vi "Autonomous Independent.vi"() -> ()   [LabVIEW 2014]
doc: "This VI is called when autonomous begins, and will automatically be terminated when autonomous ends. You can carry out timed or sensor driven robot movement independently without needing to return to the caller."
uses:
  <vilib>/Rock Robotics/WPI/DriverStation/WPI_DriverStationRobotMode2.ctl
  <vilib>/Rock Robotics/WPI/RobotDrive/WPI_RobotDriveGetSetRefNum.vi
  <vilib>/Rock Robotics/Network Tables/SD Write Numeric Array.vi
  <vilib>/Rock Robotics/WPI/RobotDrive/WPI_RobotDriveArcadeDrive_Standard(NoSaturation).vi
panel:
  out "Current Movement, for debugging":T1 {"Y Joystick Value" scale=1.0..-1.0; "X Joystick Value" scale=-1.0..1.0}
  in  "Array of robot movements":T2(array[cluster]) {"Y Joystick Value" scale=1.0..-1.0; "X Joystick Value" scale=-1.0..1.0}
  # "Be sure to right-click and choose Data Operations>>Make Current Value default if you want to save the array values with the VI"
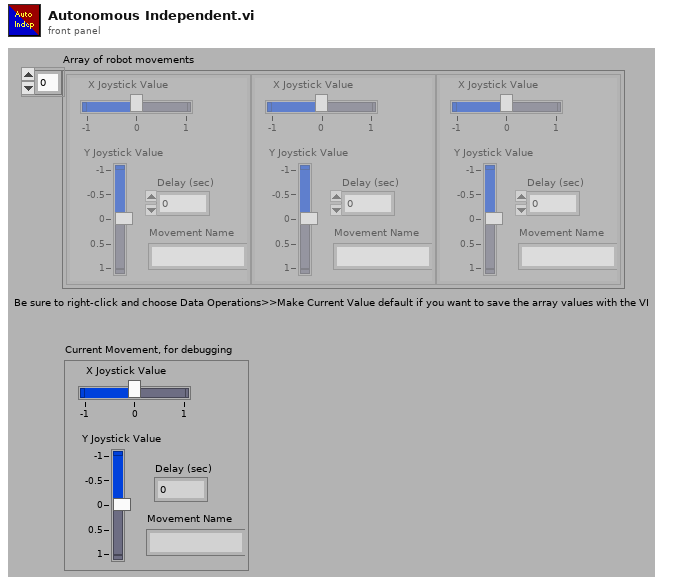
[diagram p1: front panel]
types:
  T1 = cluster{"X Joystick Value":dbl, "Y Joystick Value":dbl, "Delay (sec)":dbl, "Movement Name":string}
  T2 = cluster{"X Joystick Value":dbl, "Y Joystick Value":dbl, "Delay (sec)":dbl, "Movement Name":string}[]
  T3 = typedef "WPI_DriverStationRobotMode2.ctl" = enum16{"Autonomous Disabled", "Autonomous Enabled", "Teleop Disabled", "Teleop Enabled", "Disconnected", "Finish", "Test Disabled", "Test Enabled", "Emergency Stopped"}
  T4 = typedef "WPI_RobotDriveDevRef.ctl" = cluster{"DevStatus":errorcluster, "Motors[]":T5[], "Square Inputs":bool, "Max Output":dbl}
  T5 = typedef "WPI_MotorControlDeviceRef.ctl" = cluster{"DeviceStatus":errorcluster, "Type":T6, "PWM":cluster{"Controller":T7, "PWM Channel":T8, "DeadBand":T9}, "CAN":cluster{"Device Number":u8, "Control Mode":T10, "Semaphore":T11, "Max Vout":dbl, "TalonSRX Control Mode":T12}, "Invert":bool, "TransformRef":T13, "InvTransformRef":T13}
  T6 = typedef "WPI_MotorControlType.ctl" = enum16{"PWM", "CAN", "CANTalonSRX"}
  T7 = typedef "FPGA_TypedefDigitalModule.ctl" = enum16{"Controller 1"}
  T8 = typedef "FPGA_DIOPWMChannel.ctl" = enum8{"PWM 0", "PWM 1", "PWM 2", "PWM 3", "PWM 4", "PWM 5", "PWM 6", "PWM 7", "PWM 8", "PWM 9", "PWM MXP 0", "PWM MXP 1", "PWM MXP 2", "PWM MXP 3", "PWM MXP 4", "PWM MXP 5", "PWM MXP 6", "PWM MXP 7", "PWM MXP 8", "PWM MXP 9", "Invalid"}
  T9 = typedef "WPI_PWMDeadband.ctl" = cluster{"Name":string, "maxPositivePwm":i32, "minPositivePwm":i32, "centerPwm":i32, "maxNegativePwm":i32, "minNegativePwm":i32, "angularRange":u16}
  T10 = typedef "WPI_CANJaguar_ControlMode.ctl" = enum8{"Percent VBus", "Current", "Speed", "Position", "Voltage"}
  T11 = typedef "Semaphore RefNum" = refnum<k1>
  T12 = typedef "WPI_CANTalonSRX_APIControlMode.ctl" = enum8{"Percent VBus", "Speed", "Position", "Slave", "Unchanged / Invalid"}
  T13 = typedef "WPI_PWMTransform_ConPane.ctl" = refnum<vi>
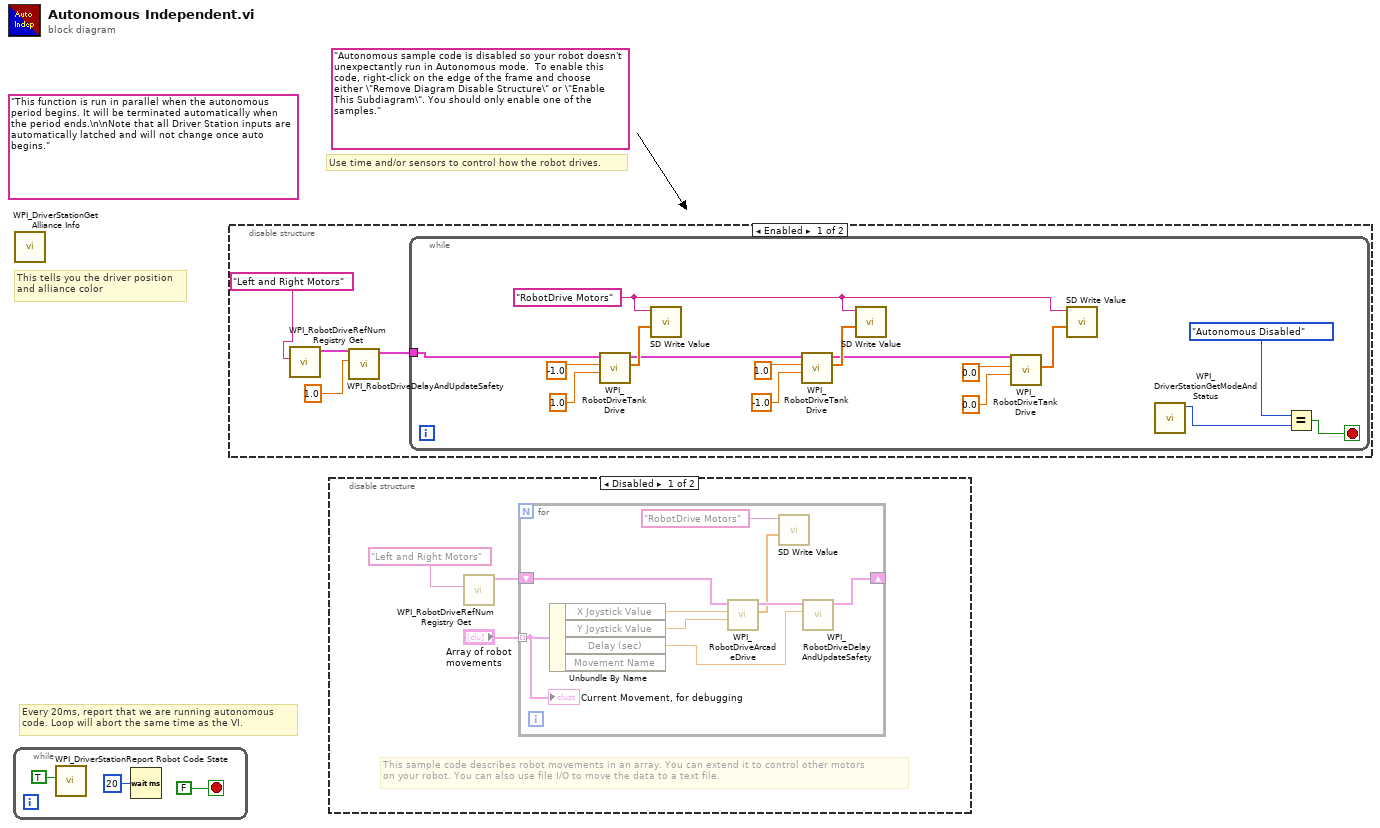
[diagram p0: block diagram]
diagram:
  (unwired) "Autonomous sample code is disabled so your robot doesn't unexpectantly run in Autonomous mode.  To enable this code, right-click on the edge of the frame and choose either \"Remove Diagram Disable Structure\" or \"Enable This Subdiagram\". You should only enable one of the samples."
  (unwired) "This function is run in parallel when the autonomous period begins. It will be terminated automatically when the period ends.\n\nNote that all Driver Station inputs are automatically latched and will not change once auto begins."
  # "Every 20ms, report that we are running autonomous\ncode. Loop will abort the same time as the VI."
  # "Use time and/or sensors to control how the robot drives."
  # "This tells you the driver position\nand alliance color"
  n1 = while {
    stop <- FALSE stop-if-true
    n2 = call <vilib>:"WPI_DriverStationReport Robot Code State.vi"("Autonomous"=TRUE) -> ()  [unwired: 10 in, 1 out]
    n3 = Wait (ms)(milliseconds to wait=u32 20) -> ()  [unwired: 1 out]
  }
  n4 = call <vilib>:"WPI_DriverStationGet Alliance Info.vi"() -> ()  [unwired: 12 out]
  n5 = disable-structure shown="Enabled" {
    frame Enabled {
      n6 = call <vilib>:"WPI_RobotDriveRefNum Registry Get.vi"("refnum name"="Left and Right Motors") -> ("RobotDriveDevRef"=w5:T4)  [unwired: 1 in, 9 out]
      n7 = call <vilib>:"WPI_RobotDriveDelayAndUpdateSafety.vi"("Delay (s)"=1.0, "RobotDriveDevRef"=w5) -> ("RobotDriveDevRef 2"=w4:T4)  [unwired: 8 in, 1 out]
      n8 = while {
        tunnel: w4 -> [w10]
        stop <- w11 stop-if-true
        w17 = "RobotDrive Motors" ("Name")
        n9 = call <vilib>:"WPI_RobotDriveTankDrive.vi"("Right axis value"=1.0 ("X axis value"), "Left axis value"=-1.0 ("X axis value"), "RobotDriveDevRef"=w10) -> ("Motor Values"=w16:dbl[], "RobotDriveDevRef"=w9:T4)  [unwired: 6 in, 1 out]
        n10 = call-poly <vilib>:"SD Write Value.vi"("Numeric Array"=w16, "Name"=w17) -> ()  [unwired: 8 in, 2 out]
        n11 = call <vilib>:"WPI_RobotDriveTankDrive.vi"("Right axis value"=-1.0 ("X axis value"), "Left axis value"=1.0 ("X axis value"), "RobotDriveDevRef"=w9) -> ("Motor Values"=w15:dbl[], "RobotDriveDevRef"=w8:T4)  [unwired: 6 in, 1 out]
        n12 = call-poly <vilib>:"SD Write Value.vi"("Numeric Array"=w15, "Name"=w17) -> ()  [unwired: 8 in, 2 out]
        n13 = call <vilib>:"WPI_RobotDriveTankDrive.vi"("Right axis value"=0.0 ("X axis value"), "Left axis value"=0.0 ("X axis value"), "RobotDriveDevRef"=w8) -> ("Motor Values"=w14:dbl[])  [unwired: 6 in, 2 out]
        n14 = call-poly <vilib>:"SD Write Value.vi"("Numeric Array"=w14, "Name"=w17) -> ()  [unwired: 8 in, 2 out]
        n15 = call <vilib>:"WPI_DriverStationGetModeAndStatus.vi"() -> ("Robot Mode"=w12:T3)  [unwired: 10 in, 1 out]
        n16 = Equal?(x=WPI_DriverStationRobotMode2."Autonomous Disabled" ("Robot Mode"), y=w12) -> (x = y?=w11:bool)
      }
    }
    frame Disabled {
    }
  }
  n17 = disable-structure shown="Disabled" {
    frame Disabled {
      # "This sample code describes robot movements in an array. You can extend it to control other motors\non your robot. You can also use file I/O to move the data to a text file."
      n18 = call <vilib>:"WPI_RobotDriveRefNum Registry Get.vi"("refnum name"="Left and Right Motors") -> ("RobotDriveDevRef"=w25:T4)  [unwired: 1 in, 9 out]
      n19 = for {
        shift-right: [w32] -> _
        shift-left: w25 -> [w33]
        tunnel: "Array of robot movements" -> [w28] mode=indexing
        n20 = Unbundle By Name(w28) -> ("X Joystick Value"=w31:dbl, "Y Joystick Value"=w30:dbl, "Delay (sec)"=w29:dbl)  [unwired: 1 out]
        n21 = call-poly <vilib>:"WPI_RobotDriveArcadeDrive.vi"("Y axis value"=w30, "X axis value"=w31, "RobotDriveDevRef"=w33) -> ("Motor Values"=w27:dbl[], "RobotDriveDevRef"=w34:T4)  [unwired: 1 in, 6 out]
        n22 = call-poly <vilib>:"SD Write Value.vi"("Numeric Array"=w27, "Name"="RobotDrive Motors") -> ()  [unwired: 8 in, 2 out]
        n23 = call <vilib>:"WPI_RobotDriveDelayAndUpdateSafety.vi"("Delay (s)"=w29, "RobotDriveDevRef"=w34) -> ("RobotDriveDevRef 2"=w32:T4)  [unwired: 8 in, 1 out]
        "Current Movement, for debugging" <- w28
      }
    }
    frame Enabled {
    }
  }
